vi "DCA Retrieve Key Array for Config.vi"(8 "error in (no error)":errorcluster, 10 "Key Array In":T13, 11 "Connection Refnum":T1) -> (0 "error out":errorcluster, 2 "DCA Test Parameters":T2={"Stimulus"={"Use Instrument"=FALSE, "Normalize"=FALSE, "Blank Screen"=FALSE, "Measurement Type"=enum."Diode", "Range"=enum."Auto", "Resolution"=enum."Auto"}, "Measurement"={"Topology"=enum."PI-Network", "Lock Topology"=FALSE, "ATTN Calc"=enum."Power", "Zo"=50.0}, "Limits"=[], "Normalization"={"Normalized?"=FALSE, "Rab Value"=0.0, "Rac Value"=0.0, "Rbc Value"=0.0}}, 3 "Connection Refnum":T1)   [LabVIEW 2011]
uses:
  ITK EXT/utils/keyedarr.llb/Keyed Array.ctl
  TypeDefs/DCA Test Parameters.ctl
  TypeDefs/DCA Stimulus Parameters.ctl
  TypeDefs/DCA Measurement Cluster.ctl
  TypeDefs/DCA Topology.ctl
  TypeDefs/DCA Attenuation Calculation.ctl
  TypeDefs/DCA Limit.ctl
  TypeDefs/DCA Limit Quantity.ctl
  TypeDefs/DCA Limit Comparison.ctl
  TypeDefs/DCA Limit Operation.ctl
  Test Referential Limit.ctl
  TypeDefs/DCA Calibration State.ctl
  Summitek EXT/ODBC/SQL Controls/Connection Refnum.ctl
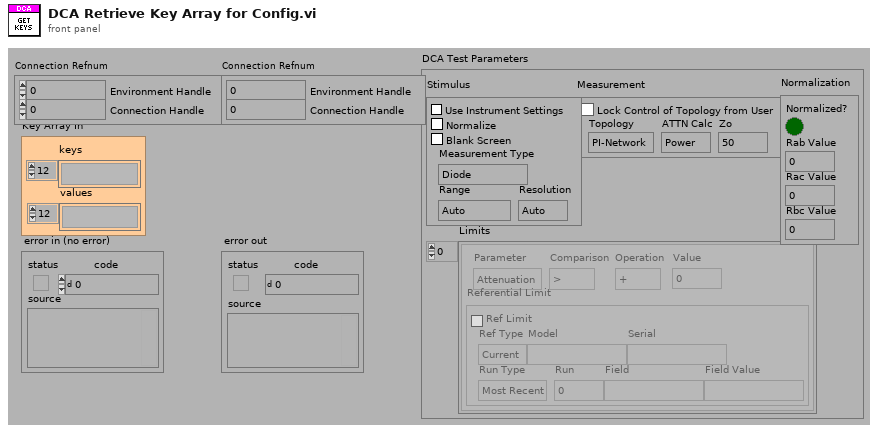
[diagram p1: front panel]
types:
  T1 = typedef "Connection Refnum.ctl" = cluster{"Environment Handle":i32, "Connection Handle":i32}
  T2 = typedef "DCA Test Parameters.ctl" = cluster{"Stimulus":T3, "Measurement":T4, "Limits":T7[], "Normalization":T12}
  T3 = typedef "DCA Stimulus Parameters.ctl" = cluster{"Use Instrument":bool, "Normalize":bool, "Blank Screen":bool, "Measurement Type":enum16{"Voltage DC", "Voltage DC Ratio", "Voltage AC", "Current DC", "Current AC", "Resistance", "Fresistance", "Frequency", "Period", "Continuity", "Diode"}, "Range":enum16{"Auto", "Minimum", "Maximum", "100", "1,000", "10,000", "100,000", "1,000,000", "10,000,000", "100,000,000"}, "Resolution":enum16{"Auto", "4 1/2", "5 1/2", "6 1/2"}}
  T4 = typedef "DCA Measurement Cluster.ctl" = cluster{"Topology":T5, "Lock Topology":bool, "ATTN Calc":T6, "Zo":dbl}
  T5 = typedef "DCA Topology.ctl" = enum32{"PI-Network", "T-Network"}
  T6 = typedef "DCA Attenuation Calculation.ctl" = enum32{"Power", "Voltage"}
  T7 = typedef "DCA Limit.ctl" = cluster{"Parameter":T8, "Comparison":T9, "Operation":T10, "Value":dbl, "Referential Limit":T11}
  T8 = typedef "DCA Limit Quantity.ctl" = enum16{"Attenuation", "Zin", "Zout", "R1", "R2", "R3", "Rab", "Rac", "Rbc"}
  T9 = typedef "DCA Limit Comparison.ctl" = enum16{">", ">=", "<", "<="}
  T10 = typedef "DCA Limit Operation.ctl" = enum16{"+", "-"}
  T11 = typedef "Test Referential Limit.ctl" = cluster{"Ref Limit":bool, "Ref Type":enum16{"Current", "Specify"}, "Model":string, "Serial":string, "Run Type":enum16{"Most Recent", "Run #", "Match Field"}, "Run":i32, "Field":string, "Field Value":string}
  T12 = typedef "DCA Calibration State.ctl" = cluster{"Normalized?":bool, "Rab Value":dbl, "Rac Value":dbl, "Rbc Value":dbl}
  T13 = typedef "Keyed Array.ctl" = cluster{"keys":string[], "values":string[]}
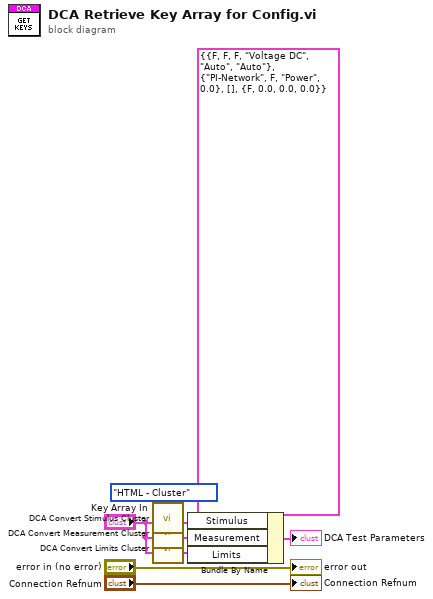
[diagram p0: block diagram]
diagram:
  w1 = enum16{"Cluster - HTML", "HTML - Cluster"}."HTML - Cluster" ("Conversion")
  n1 = call "DCA Convert Stimulus Cluster.vi"("Conversion"=w1, "Stimulus Key Array In"="Key Array In") -> ("Stimulus Cluster Out"=w3:T3)  [unwired: 1 in, 5 out]
  n2 = call "DCA Convert Measurement Cluster.vi"("Conversion"=w1, "Measurements Key Array In"="Key Array In") -> ("Measurements Cluster Out"=w5:T4)  [unwired: 1 in, 5 out]
  n3 = call "DCA Convert Limits Cluster.vi"("Conversion"=w1, "Limits Key Array In"="Key Array In") -> ("Limits Cluster Out"=w4:T7[])  [unwired: 2 in, 5 out]
  n4 = Bundle By Name(cluster=T2 {"Stimulus"={"Use Instrument"=FALSE, "Normalize"=FALSE, "Blank Screen"=FALSE, "Measurement Type"=enum."Voltage DC", "Range"=enum."Auto", "Resolution"=enum."Auto"}, "Measurement"={"Topology"=enum."PI-Network", "Lock Topology"=FALSE, "ATTN Calc"=enum."Power", "Zo"=0.0}, "Limits"=[], "Normalization"={"Normalized?"=FALSE, "Rab Value"=0.0, "Rac Value"=0.0, "Rbc Value"=0.0}} ("DCA Test Parameters"), "Stimulus"=w3, "Measurement"=w5, "Limits"=w4) -> (→"DCA Test Parameters":T2)
  "error out" <- "error in (no error)"
  "Connection Refnum" <- "Connection Refnum"
